vi "Begin.vi"(8 "error in (no error)":errorcluster, 11 "Comp XBox One Controller in":refnum<class "Comp XBox One Controller.lvclass">) -> (0 "error out":errorcluster, 3 "Comp XBox One Controller out":refnum<class "Comp XBox One Controller.lvclass">)   [LabVIEW 2014, in "Comp XBox One Controller.lvlib" / "Comp XBox One Controller.lvclass"]
uses:
  Comp XBox One Controller.lvclass
  Comp XBox One Controller.lvclass/Comp XBox One Controller.ctl
  Robot/Xbox One Controller/XBox One Controller Class/XBox One Controller.lvclass
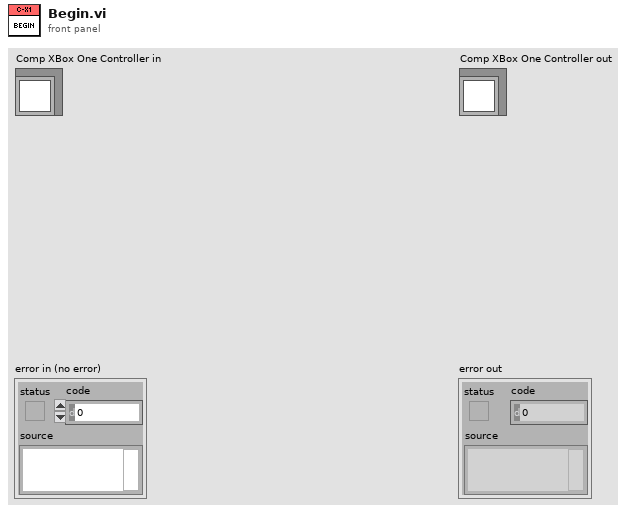
[diagram p1: front panel]
types:
  T1 = enum16{"Critical", "Error", "Warning", "Informational", "Debug"}
  T2 = typedef "WPI_JoystickDeviceEnum.ctl" = enum16{"USB 0", "USB 1", "USB 2", "USB 3", "USB 4", "USB 5"}
  T3 = typedef "WPI_JoystickDevRef.ctl" = cluster{"Device":T2}
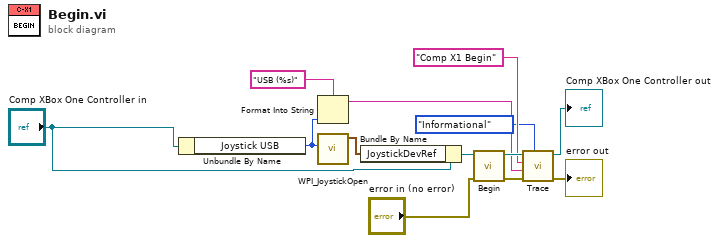
[diagram p0: block diagram]
diagram:
  n1 = Unbundle By Name("Comp XBox One Controller in") -> ("Joystick USB"=w2:T2)
  n2 = Format Into String(format string="USB (%s)", w2) -> (resulting string=w5:string)  [unwired: 2 in, 1 out]
  n3 = call <vilib>:"WPI_JoystickOpen.vi"("JoystickDevice"=w2) -> ("JoystickDevRef"=w11:T3)  [unwired: 10 in]
  n4 = Bundle By Name(cluster="Comp XBox One Controller in", "JoystickDevRef"=w11) -> (w10:refnum<class "Comp XBox One Controller.lvclass">)
  n5 = call-parent "Begin.vi"("error in (no error)"="error in (no error)", "System Actor in"=w10) -> ("error out"=w9:errorcluster, "System Actor out"=w7:refnum<class "Comp XBox One Controller.lvclass">)  [unwired: 8 in]
  n6 = call-dynamic "Trace.vi"("Trace Level"=T1."Informational", "error in (no error)"=w9, "System Message"=w5, "System Action"="Comp X1 Begin", "System Actor in"=w7) -> ("error out"=→"error out":errorcluster, "System Actor out"=→"Comp XBox One Controller out":refnum<class "Comp XBox One Controller.lvclass">)  [unwired: 5 in]
